vi "Reset Configuration.vi"(8 "error in":errorcluster, 11 "EMS Generic in":refnum<class "EMS Generic.lvclass">) -> (0 "error out":errorcluster, 3 "EMS Generic out":refnum<class "EMS Generic.lvclass">)   [LabVIEW 2018, in "EMS Generic Actor.lvlib" / "EMS Generic.lvclass"]
uses:
  EMS Generic.lvclass
  Controls/Global Configuration.ctl
  <vilib>/ORNL/CSEISMIC DDS/CSEISMIC DDS Base/Data Types/Controls/DeviceID.ctl
  <vilib>/ORNL/CSEISMIC DDS/CSEISMIC DDS Base/CSEISMIC DDS.lvclass
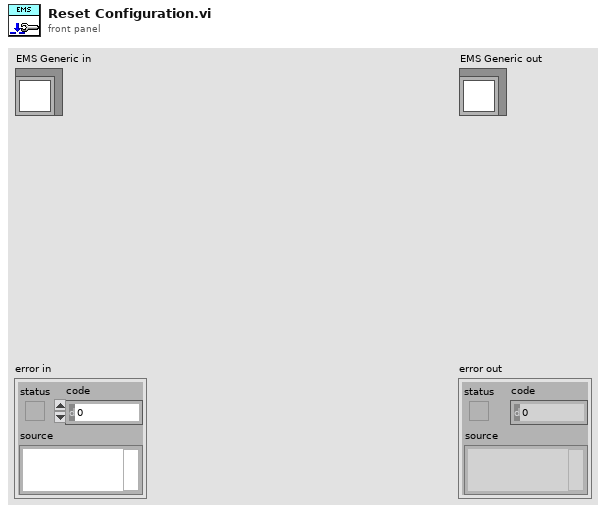
[diagram p1: front panel]
types:
  T1 = typedef "EMS Generic Actor.lvlib/EMS Generic.lvclass/Global Configuration.ctl" = cluster{"Microgrid ID":u8, "VF Device ID":T2, "Ongrid VF Priority":T2[], "Offgrid VF Priority":T2[], "AutoSwap Offgrid VF":u32, "AutoSwap Offgrid VF Delay (sec)":dbl, "AutoSwap Resynch VF":u32, "PCC Device ID":T2, "Device ID Array":T2[], "Nominal Voltage":dbl, "Nominal Frequency":dbl, "Resynch Timeout (sec)":dbl, "Island VF Activate Timeout (sec)":dbl, "Island PCC Target Power (kW)":dbl, "Island PCC Target Power Timeout (sec)":dbl, "Island Grid Settle Time (sec)":dbl, "Island PCC Failure Timeout (sec)":dbl, "Activation Devices Present Timeout (sec)":dbl, "Activation Devices Activated Timeout (sec)":dbl, "Blackstart VF GenMode Wait (sec)":dbl, "Blackstart VF DERCtrl Wait (sec)":dbl, "Blackstart Success Wait (sec)":dbl, "OnGrid Optimization Delay (sec)":dbl, "OffGrid Optimization Delay (sec)":dbl, "Resynch Frequency (Hz)":dbl, "Optimization Path":string}
  T2 = typedef "CSEISMIC DDS.lvlib/CSEISMIC DDS.lvclass/DeviceID.ctl" = string
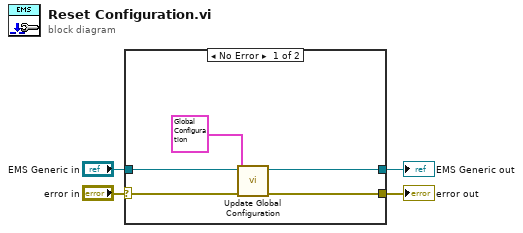
[diagram p0: block diagram]
diagram:
  n1 = case shown="No Error" "error in" {
    selector: "error in" -> [w8 w11]
    tunnel: [w7 w11] -> w3
    tunnel: [w6 w10] -> w1
    tunnel: "EMS Generic in" -> [w9 w10]
    frame No Error {
      n2 = call "Update Global Configuration.vi"("error in (no error)"=w8, "Global Configuration"=T1 {"Microgrid ID"=1, "VF Device ID"="", "Ongrid VF Priority"=[], "Offgrid VF Priority"=[], "AutoSwap Offgrid VF"=0, "AutoSwap Offgrid VF Delay (sec)"=0.0, "AutoSwap Resynch VF"=0, "PCC Device ID"="", "Device ID Array"=[], "Nominal Voltage"=0.0, "Nominal Frequency"=0.0, "Resynch Timeout (sec)"=0.0, "Island VF Activate Timeout (sec)"=0.0, "Island PCC Target Power (kW)"=0.0, "Island PCC Target Power Timeout (sec)"=0.0, "Island Grid Settle Time (sec)"=0.0, "Island PCC Failure Timeout (sec)"=0.0, "Activation Devices Present Timeout (sec)"=0.0, "Activation Devices Activated Timeout (sec)"=0.0, "Blackstart VF GenMode Wait (sec)"=0.0, "Blackstart VF DERCtrl Wait (sec)"=0.0, "Blackstart Success Wait (sec)"=0.0, "OnGrid Optimization Delay (sec)"=0.0, "OffGrid Optimization Delay (sec)"=0.0, "Resynch Frequency (Hz)"=0.0, "Optimization Path"=""}, "EMS Generic in"=w9) -> ("error out"=w7:errorcluster, "EMS Generic out"=w6:refnum<class "EMS Generic.lvclass">)  [unwired: 7 in]
    }
    frame Error {
    }
  }
  "error out" <- w3
  "EMS Generic out" <- w1
